vi "GV pockels delay.vi"() -> ()   [LabVIEW 2017]
panel:
  out "PockelsDelay_tick":u16
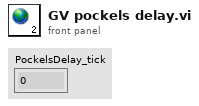
[diagram p1: front panel]
diagram:
